vi "Test Yahoo - URL - Build (for stock ticker) - 01.vi"(8 "error in (no error)":errorcluster, 11 "TestCase in":refnum<class "TestCase.lvclass">) -> (0 "error out":errorcluster, 3 "TestCase out":refnum<class "TestCase.lvclass">)   [LabVIEW 2011, in "test.lvclass"]
uses:
  test.lvclass
  <vilib>/addons/_JKI Toolkits/VI Tester/TestCase.llb/TestCase.lvclass
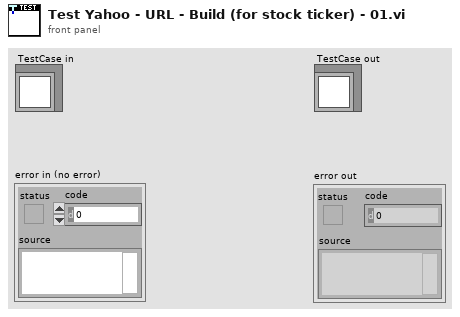
[diagram p1: front panel]
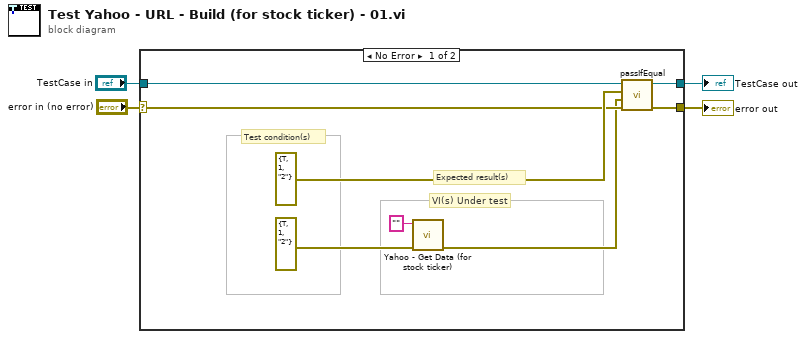
[diagram p0: block diagram]
diagram:
  n1 = case shown="No Error" "error in (no error)" {
    selector: "error in (no error)" -> [w8 w13]
    tunnel: "TestCase in" -> [w9 w14]
    tunnel: [w7 w14] -> w3
    tunnel: [w6 w13] -> w2
    frame No Error {
      # "Expected result(s)"
      # "Test condition(s)"
      # "VI(s) Under test"
      n2 = call "Yahoo - Get Data (for stock ticker).vi"("Symbol"="", "error in"=errorcluster {"status"=TRUE, "code"=1, "source"="2"} ("error in (no error)")) -> ("error out"=w5:errorcluster)  [unwired: 6 in, 1 out]
      n3 = call-dynamic "passIfEqual.vi"("error in (no error)"=w8, "y"=w5, "x"=errorcluster {"status"=TRUE, "code"=1, "source"="2"} ("error in (no error)"), "TestCase in"=w9) -> ("error out"=w6:errorcluster, "TestCase out"=w7:refnum<class "TestCase.lvclass">)  [unwired: 6 in]
    }
    frame Error {
    }
  }
  "TestCase out" <- w3
  "error out" <- w2
